vi "RTAF Global References.vi"() -> ()   [LabVIEW 2020]
uses:
  Logger/API/Logger Actor API.lvclass
  Alarms Handler/API/Alarms Handler Actor API.lvclass
  Test/API/Test Actor API.lvclass
panel:
  in  "Test":refnum<class "Test Actor API.lvclass">
  in  "Alarms Handler":refnum<class "Alarms Handler Actor API.lvclass">
  in  "Logger":refnum<class "Logger Actor API.lvclass">
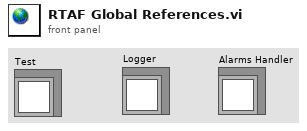
[diagram p1: front panel]
diagram:
